vi "Encoder Config Pane.vi"(6 "_SubPanelMessages":refnum<notifier>, 9 "_myEmbeddedToFrameEvent":T5, 10 "_myEmbedded.Exit":refnum<user-event>, 11 "_Property Bundle":cluster{"Name":string, "Value":variant}[](array[cluster])) -> (1 "_Connection Informations":T1, 2 "_Scripter Input":T7)   [LabVIEW 2021]
doc: "Reads and decodes signals from an encoder. This Express VI reads the number of ticks that the encoder receives since the last counter reset."
uses:
  <vilib>/myRIO/Common/Express VI Framework/xctls/myRIO Channel Name/myRIO Channel Name.xctl
  <vilib>/myRIO/Common/Express VI Framework/typedefs/Config Pane to Framework Ref.ctl
  <vilib>/myRIO/Common/Express VI Framework/typedefs/Data Validate Ref.ctl
  <vilib>/myRIO/Common/Express VI Framework/typedefs/Scripter Input.ctl
  <vilib>/myRIO/Common/Express VI Framework/typedefs/WireThrough Terminal Names.ctl
  <vilib>/myRIO/Common/Express VI Framework/typedefs/Instrument Driver Method Descriptor Array.ctl
  <vilib>/myRIO/Common/Express VI Framework/typedefs/Instrument Driver Method Descriptor.ctl
  <vilib>/myRIO/Common/Express VI Framework/typedefs/Sub Panel Messages.ctl
  <vilib>/myRIO/Common/Express VI Framework/typedefs/Connection Informations.ctl
  <vilib>/myRIO/Common/Instrument Driver Framework/Utilities/typedefs/Channel Types.ctl
  <vilib>/myRIO/Common/Instrument Driver Framework/myRIO v1.0/Encoder/typedefs/Encoder Signal Mode.ctl
panel:
  in  "Encoder output signal type":enum32{"Quadrature phase", "Step and direction"}(radio) caption="Encoder output signal type:"
  out "_Channel Details:":string caption="Connections:"
  in  "Channel:":u16(xcontrol)
  in  "_Default Alias String":string
  in  "_VI Default Name (Edit and make value default)":string="Encoder"
  in  "Name:":string caption="Node name:"
  in  "_WireThrough Info (Edit and make value default)":T2={"WireThrough Top In"="Encoder Ref In", "WireThrough Bottom In"="error in (no error)", "WireThrough Top Out"="Encoder Ref Out", "WireThrough Bottom Out"="error out"}
  in  "_Template Array (Edit and make value default)":T3=[{"Function Name"="Smart Open", "VI Path"=path "<vilib>/myRIO/Instrument Drivers/Onboard IO/Encoder/vis", "Script"=TRUE, "Inputs"=[{"name"="Channel Name", "value"=variant, "Config Pane Only"=TRUE, "Build Array"=FALSE, "Bundle Cluster"=FALSE, "Show Term"=FALSE, "alias"=[], "Required Input"=FALSE}, {"name"="Encoder Signal Mode", "value"=variant, "Config Pane Only"=TRUE, "Build Array"=FALSE, "Bundle Cluster"=FALSE, "Show Term"=FALSE, "alias"=[], "Required Input"=FALSE}, {"name"="Start Counter", "value"=variant, "Config Pane Only"=TRUE, "Build Array"=FALSE, "Bundle Cluster"=FALSE, "Show Term"=FALSE, "alias"=[], "Required Input"=FALSE}], "Outputs"=[], "VI Class"=enum."Open", "Controls Refs[]"=[], "Inline"=FALSE}, {"Function Name"="Open", "VI Path"=path "<vilib>/myRIO/Instrument Drivers/Onboard IO/Encoder/vis", "Script"=FALSE, "Inputs"=[{"name"="Channel Name", "value"=variant, "Config Pane Only"=TRUE, "Build Array"=FALSE, "Bundle Cluster"=FALSE, "Show Term"=FALSE, "alias"=[], "Required Input"=FALSE}, {"name"="Encoder Signal Mode", "value"=variant, "Config Pane Only"=TRUE, "Build Array"=FALSE, "Bundle Cluster"=FALSE, "Show Term"=FALSE, "alias"=[], "Required Input"=FALSE}, {"name"="Start Counter", "value"=variant, "Config Pane Only"=TRUE, "Build Array"=FALSE, "Bundle Cluster"=FALSE, "Show Term"=FALSE, "alias"=[], "Required Input"=FALSE}], "Outputs"=[], "VI Class"=enum."Open", "Controls Refs[]"=[], "Inline"=FALSE}, {"Function Name"="Read", "VI Path"=path "<vilib>/myRIO/Instrument Drivers/Onboard IO/Encoder/vis", "Script"=TRUE, "Inputs"=[{"name"="Reset Counter", "value"=variant, "Config Pane Only"=FALSE, "Build Array"=FALSE, "Bundle Cluster"=FALSE, "Show Term"=TRUE, "alias"=[], "Required Input"=FALSE}], "Outputs"=[{"name"="Counter Value", "value"=variant, "Show Term"=TRUE, "Index Array"=FALSE, "Unbundle Cluster"=FALSE, "alias"=[]}, {"name"="Counter Direction", "value"=variant, "Show Term"=TRUE, "Index Array"=FALSE, "Unbundle Cluster"=FALSE, "alias"=[]}, {"name"="Overflow?", "value"=variant, "Show Term"=TRUE, "Index Array"=FALSE, "Unbundle Cluster"=FALSE, "alias"=[]}], "VI Class"=enum."Data", "Controls Refs[]"=[], "Inline"=FALSE}, {"Function Name"="Close", "VI Path"=path "<vilib>/myRIO/Instrument Drivers/Onboard IO/Encoder/vis", "Script"=FALSE, "Inputs"=[], "Outputs"=[], "VI Class"=enum."Close", "Controls Refs[]"=[], "Inline"=FALSE}]
  in  "_Test Close":bool
  # "User Visible Area"
  # "NOTE: Tab Order has been set\nfor this Front Panel.\n\nSee Edit>>Set Tabbing Order...\n\nAll controls that are not visible at \nruntime are excluded from Tabbing order\n\nTo exlude a control from context\nhelp prefix its label text with a '-'"
  # "Most encoders generate a quadrature phase signal that can be interpreted as Gray code. Choose this option if you are not sure about the signal type of your encoder."
  # "In some cases, encoders generate a signal for step and a signal for direction."
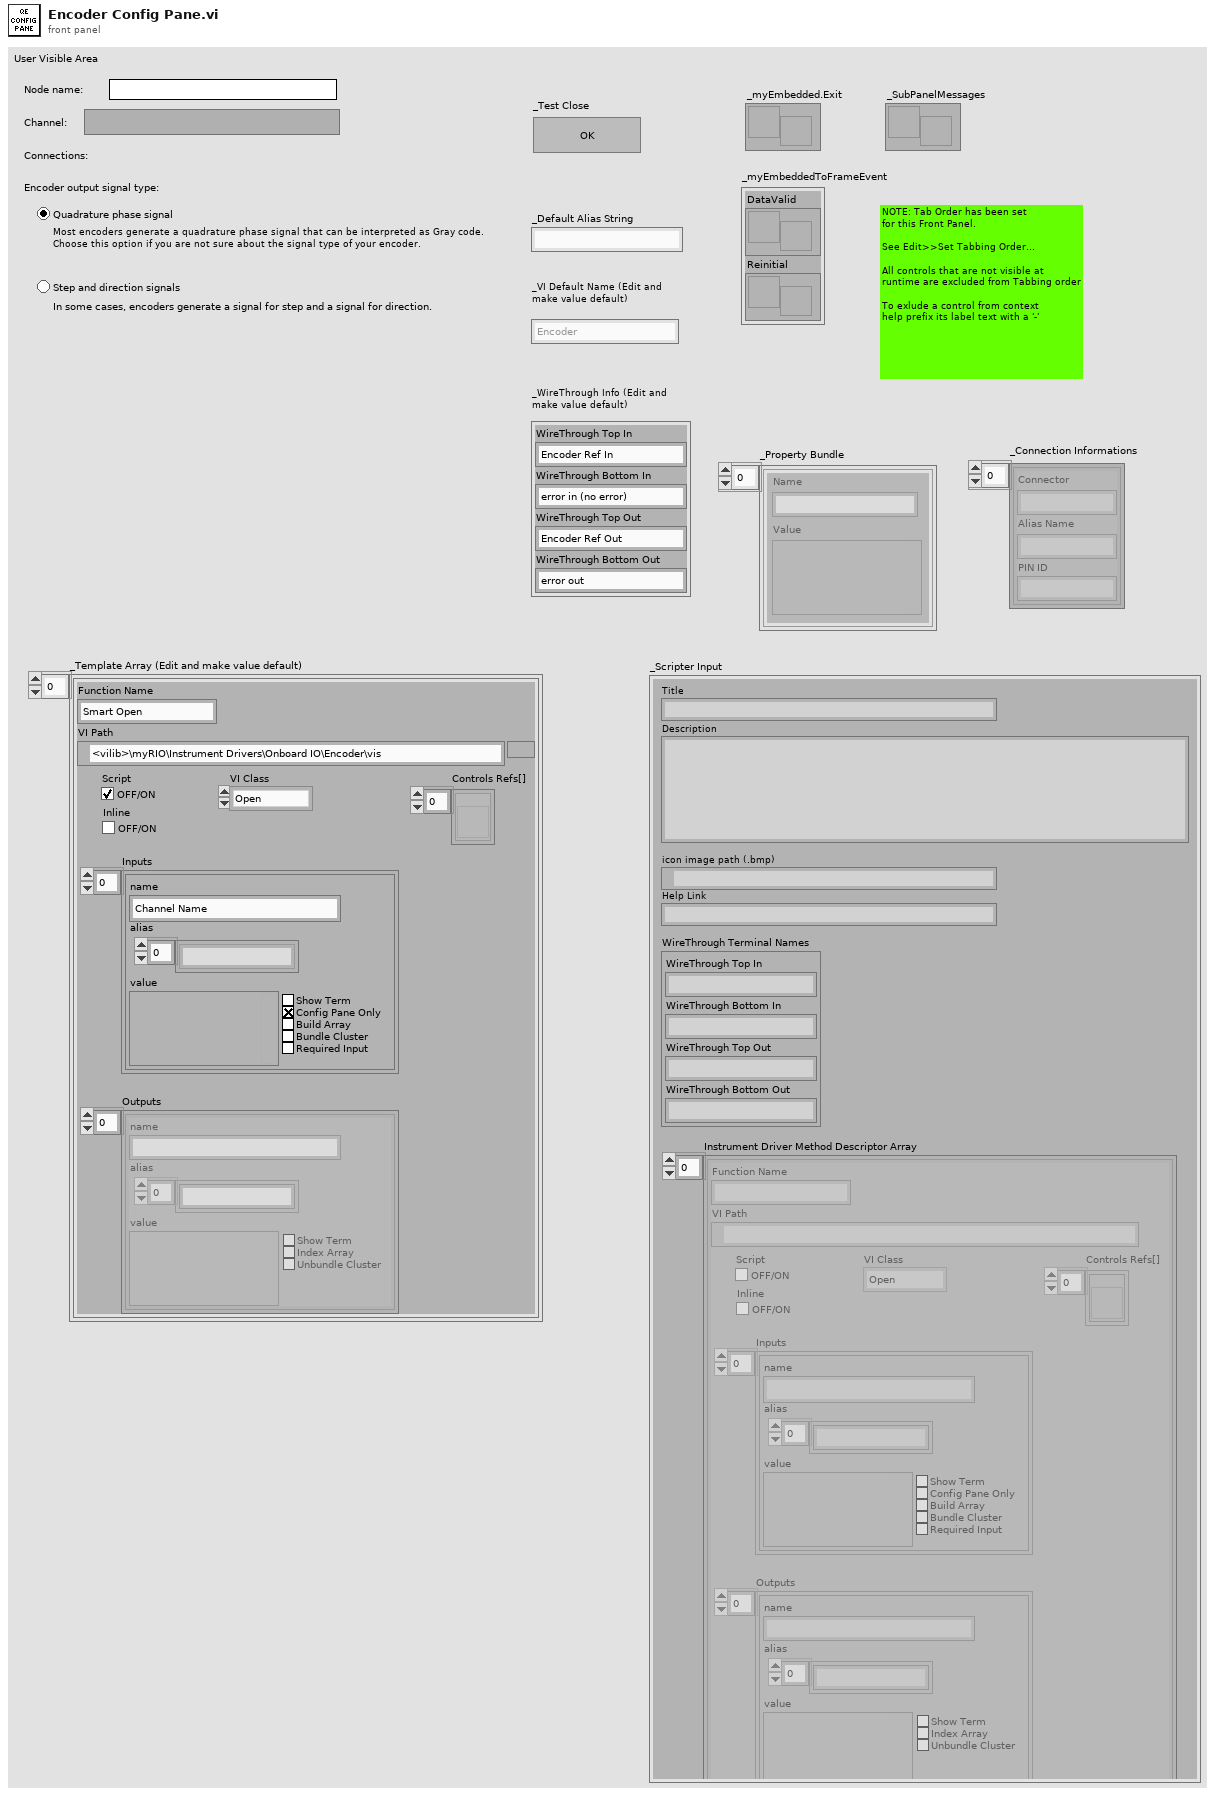
[diagram p1: front panel]
types:
  T1 = typedef "Connection Informations.ctl" = cluster{"Connector":string, "Alias Name":string, "PIN ID":string}[]
  T2 = typedef "WireThrough Terminal Names.ctl" = cluster{"WireThrough Top In":string, "WireThrough Bottom In":string, "WireThrough Top Out":string, "WireThrough Bottom Out":string}
  T3 = typedef "Instrument Driver Method Descriptor Array.ctl" = T4[]
  T4 = typedef "Instrument Driver Method Descriptor.ctl" = cluster{"Function Name":string, "VI Path":path, "Script":bool, "Inputs":cluster{"name":string, "value":variant, "Config Pane Only":bool, "Build Array":bool, "Bundle Cluster":bool, "Show Term":bool, "alias":string[], "Required Input":bool}[], "Outputs":cluster{"name":string, "value":variant, "Show Term":bool, "Index Array":bool, "Unbundle Cluster":bool, "alias":string[]}[], "VI Class":enum16{"Open", "Configure", "Data", "Manage", "Close"}, "Controls Refs[]":refnum<vi>[], "Inline":bool}
  T5 = typedef "Config Pane to Framework Ref.ctl" = cluster{"DataValid":T6, "Reinitial":refnum<user-event>}
  T6 = typedef "Data Validate Ref.ctl" = refnum<user-event>
  T7 = typedef "Scripter Input.ctl" = cluster{"Title":string, "Description":string, "icon image path (.bmp)":path, "Help Link":string, "WireThrough Terminal Names":T2, "Instrument Driver Method Descriptor Array":T3}
  T8 = typedef "Channel Types.ctl" = enum32{"Unknown", "AI", "AO", "DIO - DI", "DIO", "DIO - DO", "I2C", "PWM", "Encoder", "SPI", "UART", "Accelerometer", "DIO - LED", "DIO - Button", "AI (N Samples)", "AudioIn (N Samples)", "AO (N Samples)", "AudioOut (N Samples)", "DI (N Samples)", "DO (N Samples)", "AI IRQ", "DI IRQ", "Timer IRQ", "RSL", "Relay", "CAN", "AI (Continuous)", "AO (Continuous)"}
  T9 = typedef "Channel Info.ctl" = cluster{"Channel Name":string, "Alias":string, "Used?":bool, "Not Support?":bool, "Property Bundle":cluster{"Name":string, "Value":variant}[]}
  T10 = typedef "Sub Panel Messages.ctl" = enum16{"Initialized"}
  T11 = cluster{"Connector":string, "Alias Name":string, "PIN ID":string}
  T12 = typedef "Encoder Signal Mode.ctl" = enum16{"Quadrature phase signal", "Step and direction signal"}
  T13 = cluster{"name":string, "value":variant, "Config Pane Only":bool, "Build Array":bool, "Bundle Cluster":bool, "Show Term":bool, "alias":string[], "Required Input":bool}[]
  T14 = cluster{"name":string, "value":variant, "Config Pane Only":bool, "Build Array":bool, "Bundle Cluster":bool, "Show Term":bool, "alias":string[], "Required Input":bool}
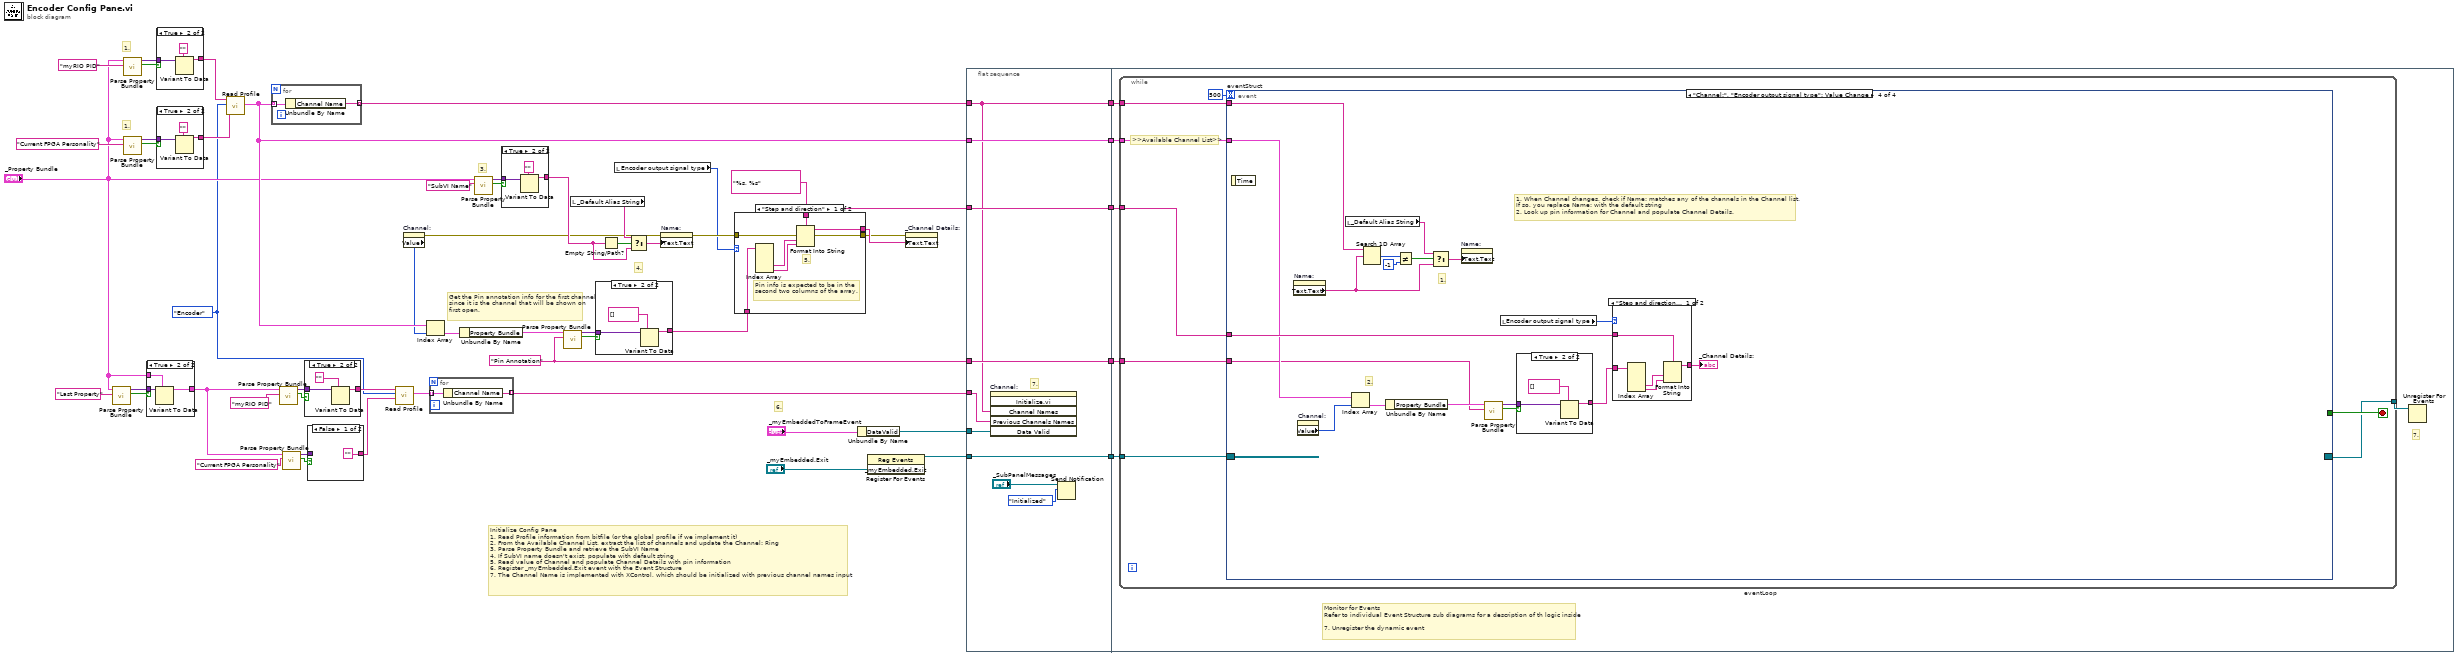
[diagram p0: block diagram]
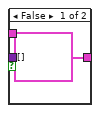
[diagram p2: hidden frame]
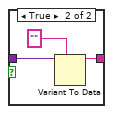
[diagram p3: hidden frame]
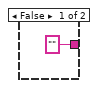
[diagram p4: hidden frame]
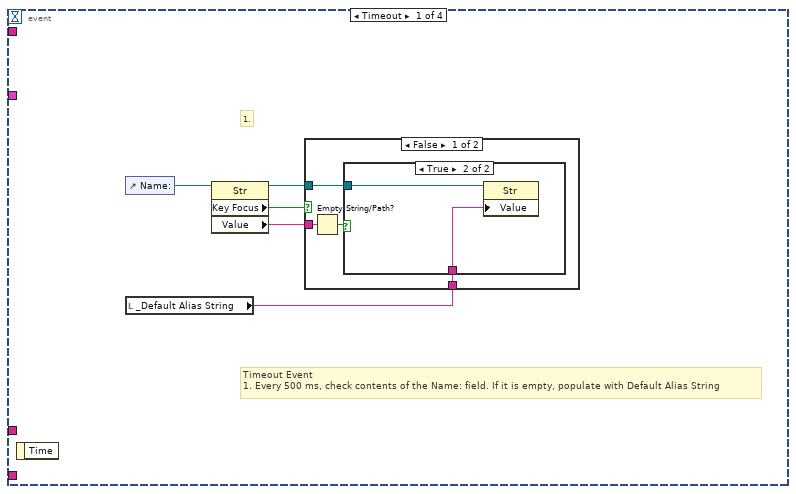
[diagram p5: hidden frame]
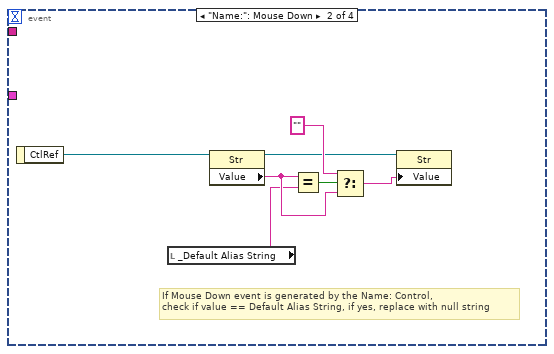
[diagram p8: hidden frame]
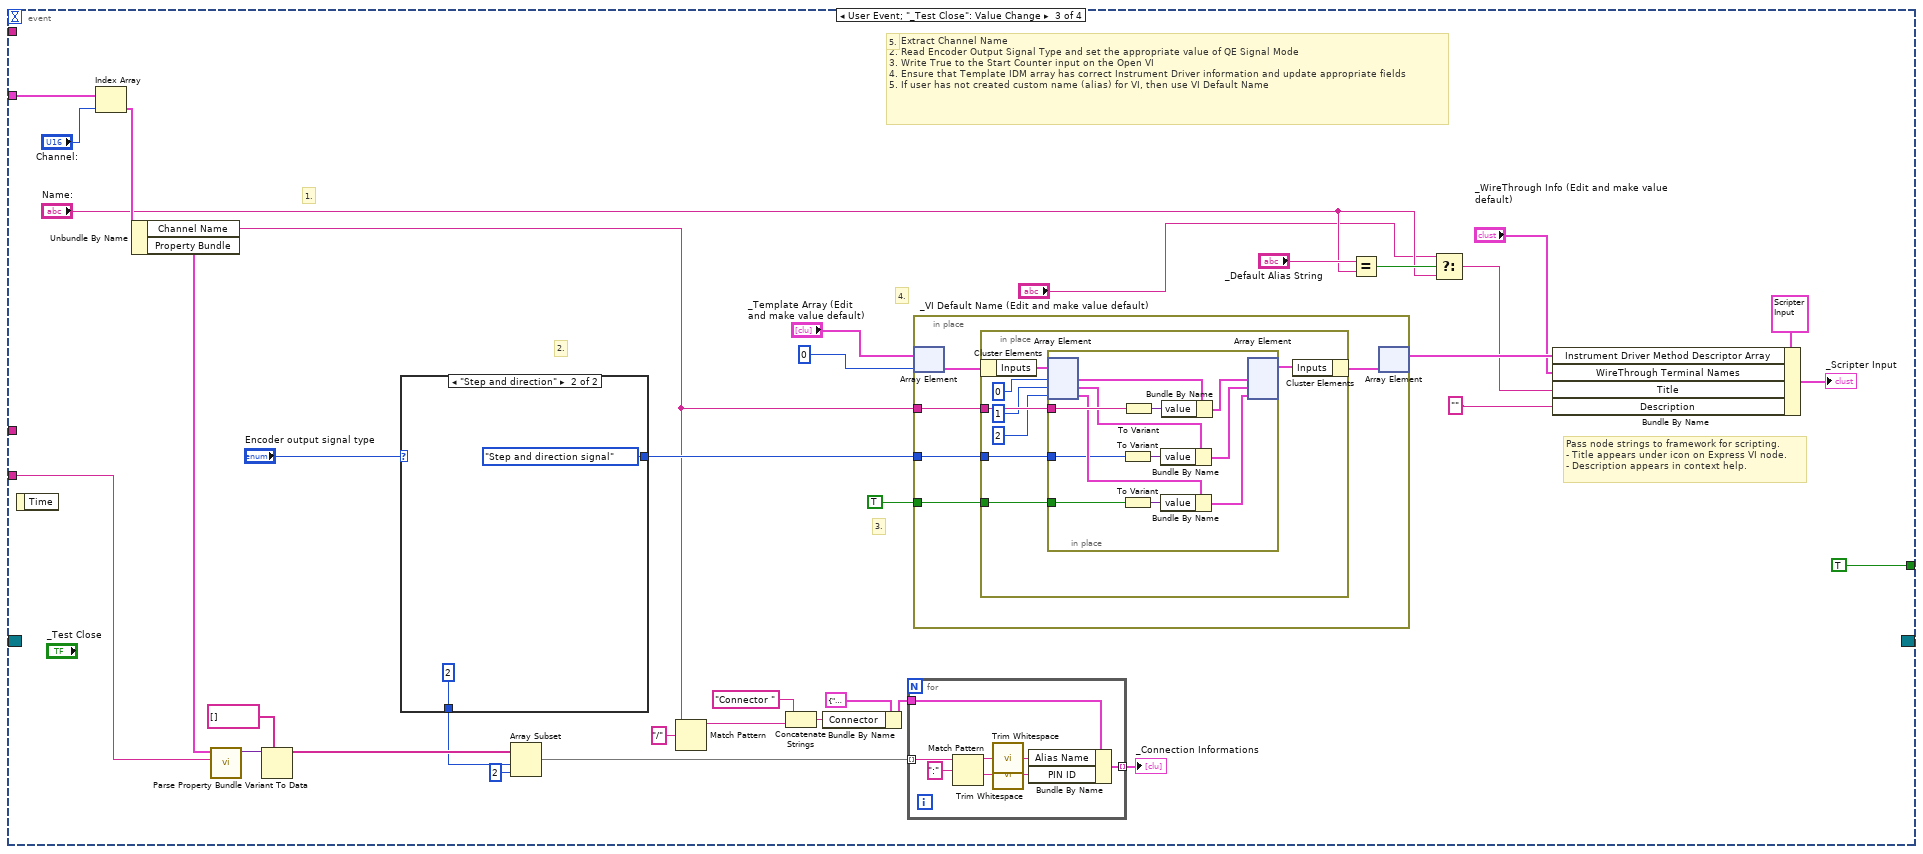
[diagram p9: hidden frame]
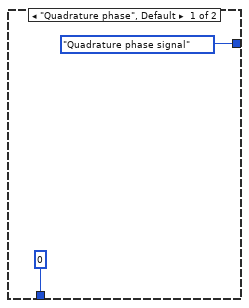
[diagram p10: hidden frame]
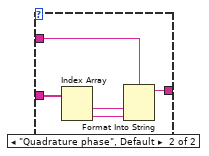
[diagram p11: hidden frame]
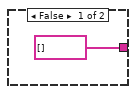
[diagram p12: hidden frame]
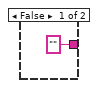
[diagram p13: hidden frame]
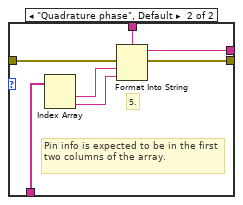
[diagram p14: hidden frame]
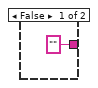
[diagram p15: hidden frame]
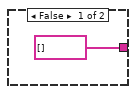
[diagram p16: hidden frame]
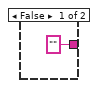
[diagram p17: hidden frame]
diagram:
  w1 = Channel_Types."Encoder" ("Channel to Read")
  w34 = "Pin Annotation" ("Name")
  w41 = "%s, %s"
  # "1."
  # "Get the Pin annotation info for the first channel  since it is the channel that will be shown on first open."
  # "1."
  # "6."
  # "4."
  # "3."
  # "Initialize Config Pane\n1. Read Profile information from bitfile (or the global profile if we implement it)\n2. From the Available Channel List, extract the list of channels and update the Channel: Ring\n3. Parse Property Bundle and retrieve the SubVI Name\n4. If SubVI name doesn't exist, populate with default string\n5. Read value of Channel and populate Channel Details with pin information \n6. Register _myEmbedded.Exit event with the Event Structure\n7. The Channel Name is implemented with XControl, which should be initialized with previous channel names input"
  n1 = call <vilib>:"Parse Property Bundle.vi"("Name"="Last Property", "Property Bundle"="_Property Bundle") -> ("Found?"=w8:bool, "Value"=w9:variant)  [unwired: 8 in]
  n2 = call <vilib>:"Parse Property Bundle.vi"("Name"="myRIO PID", "Property Bundle"="_Property Bundle") -> ("Found?"=w33:bool, "Value"=w32:variant)  [unwired: 8 in]
  n3 = call <vilib>:"Parse Property Bundle.vi"("Name"="Current FPGA Personality", "Property Bundle"="_Property Bundle") -> ("Found?"=w26:bool, "Value"=w27:variant)  [unwired: 8 in]
  n4 = case shown="True" w8 {
    tunnel: w9 -> [_ w59]
    tunnel: [cluster{"Name":string, "Value":variant}[] [] ("_Property Bundle") w58] -> w7
    tunnel: "_Property Bundle" -> [_ w57]
    frame False {
    }
    frame True {
      n5 = Variant To Data(type=w57, Variant=w59) -> (data=w58:cluster{"Name":string, "Value":variant}[])  [unwired: 1 in, 1 out]
    }
  }
  n6 = case shown="True" w33 {
    tunnel: w32 -> [_ w63]
    tunnel: ["" ("Name") w61] -> w30
    frame False {
    }
    frame True {
      n7 = Variant To Data(type="" ("Name"), Variant=w63) -> (data=w61:string)  [unwired: 1 in, 1 out]
    }
  }
  n8 = case shown="True" w26 {
    tunnel: w27 -> [_ w67]
    tunnel: ["" ("Name") w65] -> w25
    frame False {
    }
    frame True {
      n9 = Variant To Data(type="" ("Name"), Variant=w67) -> (data=w65:string)  [unwired: 1 in, 1 out]
    }
  }
  n10 = call <vilib>:"Read Profile.vi"("FPGA Name"=w25, "Channel to Read"=w1, "myRIO PID"=w30) -> ("Channel List Out"=w38:T9[])  [unwired: 7 in, 1 out]
  n11 = for {
    tunnel: [w69] -> w4 mode=indexing
    tunnel: w38 -> [w68] mode=indexing
    n12 = Unbundle By Name(w68) -> ("Channel Name"=w69:string)
  }
  n13 = call <vilib>:"Parse Property Bundle.vi"("Name"="myRIO PID", "Property Bundle"=w7) -> ("Found?"=w17:bool, "Value"=w16:variant)  [unwired: 8 in]
  n14 = call <vilib>:"Parse Property Bundle.vi"("Name"="Current FPGA Personality", "Property Bundle"=w7) -> ("Found?"=w12:bool, "Value"=w13:variant)  [unwired: 8 in]
  n15 = case shown="True" w17 {
    tunnel: w16 -> [_ w73]
    tunnel: ["" ("Name") w71] -> w18
    frame False {
    }
    frame True {
      n16 = Variant To Data(type="" ("Name"), Variant=w73) -> (data=w71:string)  [unwired: 1 in, 1 out]
    }
  }
  n17 = case shown="False" w12 {
    tunnel: w13 -> [_ w77]
    tunnel: ["" ("Name") w75] -> w11
    frame False {
    }
    frame True {
      n18 = Variant To Data(type="" ("Name"), Variant=w77) -> (data=w75:string)  [unwired: 1 in, 1 out]
    }
  }
  n19 = call <vilib>:"Read Profile.vi"("FPGA Name"=w11, "Channel to Read"=w1, "myRIO PID"=w18) -> ("Channel List Out"=w6:T9[])  [unwired: 7 in, 1 out]
  n20 = property on="Channel:" class="myRIO Channel Name (strict)"() -> (error out=w46:errorcluster, "Value"=w24:u16)  [unwired: 2 in, 1 out]
  n21 = Index Array(array=w38, index=w24) -> (element=w37:T9)
  n22 = for {
    tunnel: [w79] -> w2 mode=indexing
    tunnel: w6 -> [w78] mode=indexing
    n23 = Unbundle By Name(w78) -> ("Channel Name"=w79:string)
  }
  n24 = Unbundle By Name(w37) -> ("Property Bundle"=w36:cluster{"Name":string, "Value":variant}[])
  n25 = call <vilib>:"Parse Property Bundle.vi"("Name"="SubVI Name", "Property Bundle"="_Property Bundle") -> ("Found?"=w49:bool, "Value"=w48:variant)  [unwired: 8 in]
  n26 = case shown="True" w49 {
    tunnel: w48 -> [_ w83]
    tunnel: ["" ("Name") w81] -> w47
    frame False {
    }
    frame True {
      n27 = Variant To Data(type="" ("Name"), Variant=w83) -> (data=w81:string)  [unwired: 1 in, 1 out]
    }
  }
  n28 = call <vilib>:"Parse Property Bundle.vi"("Name"=w34, "Property Bundle"=w36) -> ("Found?"=w39:bool, "Value"=w40:variant)  [unwired: 8 in]
  n29 = local read "_Default Alias String"() -> (w51:string)
  n30 = case shown="True" w39 {
    tunnel: w40 -> [_ w87]
    tunnel: [string[] [] w86] -> w35
    frame False {
    }
    frame True {
      n31 = Variant To Data(type=string[] [], Variant=w87) -> (data=w86:string[])  [unwired: 1 in, 1 out]
    }
  }
  n32 = Empty String/Path?(string/path=w47) -> (empty?=w53:bool)
  n33 = local read "Encoder output signal type"() -> (w29:enum32{"Quadrature phase", "Step and direction"})
  n34 = Select(t=w51, s=w53, f=w47) -> (s? t:f=w52:string)
  n35 = property on="Name:" class="Str"(error in=w46, "Text.Text"=w52) -> (error out=w45:errorcluster)  [unwired: 1 in, 1 out]
  n36 = case shown="\"Step and direction\"" w29 {
    tunnel: w45 -> [w94 w101]
    tunnel: [w93 w100] -> w44
    tunnel: [w92 w99] -> w43
    tunnel: w41 -> [w91 w98]
    tunnel: w35 -> [w90 w95]
    frame "Step and direction" {
      # "Pin info is expected to be in the second two columns of the array."
      # "5."
      n37 = Index Array(array=w90) -> (element #3=w89:string, element #4=w88:string)  [unwired: 4 in, 2 out]
      n38 = Format Into String(format string=w91, error in=w94, w89, w88) -> (resulting string=w93:string, error out=w92:errorcluster)  [unwired: 1 in]
    }
    frame "Quadrature phase", Default {
      # "Pin info is expected to be in the first two columns of the array."
      # "5."
      n39 = Index Array(array=w95) -> (element #1=w97:string, element #2=w96:string)  [unwired: 2 in]
      n40 = Format Into String(format string=w98, error in=w101, w97, w96) -> (resulting string=w100:string, error out=w99:errorcluster)  [unwired: 1 in]
    }
  }
  n41 = Unbundle By Name("_myEmbeddedToFrameEvent") -> ("DataValid"=w23:T6)
  n42 = register-events("_myEmbedded.Exit") -> (reference out=w55:refnum<event-registration>)  [unwired: 2 in, 1 out]
  n43 = property on="_Channel Details:" class="Str"(error in=w43, "Text.Text"=w44) -> ()  [unwired: 1 in, 2 out]
  n44 = flat-sequence {
    tunnel: w23 -> [w104]
    tunnel: w34 -> [w107]
    tunnel: w38 -> [w108]
    tunnel: w41 -> [w109]
    tunnel: w55 -> [w110]
    tunnel: [w110] -> w22
    tunnel: [w109] -> w21
    tunnel: [w108] -> w20
    tunnel: [w107] -> w19
    tunnel: w4 -> [w103]
    tunnel: [w103] -> w3
    tunnel: w2 -> [w102]
    tunnel: w22 -> [w116]
    tunnel: w21 -> [w114]
    tunnel: w20 -> [w113]
    tunnel: w19 -> [w112]
    tunnel: w3 -> [w111]
    frame #0 {
      # "7."
      n45 = invoke on="Channel:" class="myRIO Channel Name (strict)" method="Initialize.vi"("Channel Names"=w103, "Previous Channels Names"=w102, "Data Valid"=w104) -> ()  [unwired: 3 in, 6 out]
      n46 = Send Notification(notification=Sub_Panel_Messages."Initialized", notifier="_SubPanelMessages") -> ()  [unwired: 1 in, 2 out]
    }
    frame #1 {
      # "7."
      # "Monitor for Events\nRefer to individual Event Structure sub diagrams for a description of th logic inside\n\n7. Unregister the dynamic event"
      n47 = while "eventLoop" {
        tunnel: w116 -> [w123]
        tunnel: [w122] -> w115
        tunnel: w113 -> [w120]
        tunnel: w114 -> [w119]
        tunnel: w112 -> [w118]
        tunnel: w111 -> [w117]
        stop <- w124 stop-if-true
        # ">>Available Channel List>>"
        n48 = event "eventStruct" shown="[3] \"Channel:\", \"Encoder output signal type\": Value Change" {
          selector: w123 -> [_ _ _ _]
          dyn-events: [_ _ _ _] -> w122
          timeout: 500 -> [_ _ _ _]
          tunnel: [_ _ TRUE ("_Test Close") _] -> w124
          tunnel: w120 -> [_ _ w176 w220]
          tunnel: w119 -> [_ _ _ w225]
          tunnel: w118 -> [_ _ w157 w217]
          tunnel: w117 -> [_ _ _ w215]
          event Timeout {
            # "Timeout Event\n1. Every 500 ms, check contents of the Name: field. If it is empty, populate with Default Alias String"
            # "1."
            n49 = event-data() -> ()  [unwired: 1 in, 1 out]
            n50 = control-ref of="Name:"() -> (w127:refnum<vi>)
            n51 = local read "_Default Alias String"() -> (w125:string)
            n52 = property on="Property Node" class="Str"(reference=w127) -> (reference out=w126:refnum<vi>, "Key Focus"=w128:bool, "Value"=w129:string)  [unwired: 1 in, 1 out]
            n53 = case shown="False" w128 {
              tunnel: w129 -> [w133 _]
              tunnel: w126 -> [w131 _]
              tunnel: w125 -> [w130 _]
              frame False {
                n54 = Empty String/Path?(string/path=w133) -> (empty?=w132:bool)
                n55 = case shown="True" w132 {
                  tunnel: w131 -> [_ w135]
                  tunnel: w130 -> [_ w134]
                  frame False {
                  }
                  frame True {
                    n56 = property on="Property Node" class="Str"(reference=w135, "Value"=w134) -> ()  [unwired: 1 in, 2 out]
                  }
                }
              }
              frame True {
              }
            }
          }
          event "Name:": Mouse Down {
            # "If Mouse Down event is generated by the Name: Control,\ncheck if value == Default Alias String, if yes, replace with null string"
            n57 = event-data() -> ("CtlRef"=w142:refnum<vi>)  [unwired: 1 in]
            n58 = local read "_Default Alias String"() -> (w136:string)
            n59 = property class="Str"(reference=w142) -> (reference out=w138:refnum<vi>, "Value"=w137:string)  [unwired: 1 in, 1 out]
            n60 = Equal?(x=w137, y=w136) -> (x = y?=w141:bool)
            n61 = Select(t="", s=w141, f=w137) -> (s? t:f=w139:string)
            n62 = property class="Str"(reference=w138, "Value"=w139) -> ()  [unwired: 1 in, 2 out]
          }
          event User Event; "_Test Close": Value Change {
            # "3."
            # "1."
            # "2."
            # "1. Extract Channel Name\n2. Read Encoder Output Signal Type and set the appropriate value of QE Signal Mode \n3. Write True to the Start Counter input on the Open VI \n4. Ensure that Template IDM array has correct Instrument Driver information and update appropriate fields\n5. If user has not created custom name (alias) for VI, then use VI Default Name"
            # "5."
            # "4."
            # "Pass node strings to framework for scripting.\n- Title appears under icon on Express VI node.\n- Description appears in context help."
            n63 = event-data() -> ()  [unwired: 1 in, 1 out]
            n64 = Index Array(array=w176, index="Channel:") -> (element=w165:T9)
            n65 = Unbundle By Name(w165) -> ("Channel Name"=w152:string, "Property Bundle"=w158:cluster{"Name":string, "Value":variant}[])
            n66 = call <vilib>:"Parse Property Bundle.vi"("Name"=w157, "Property Bundle"=w158) -> ("Value"=w156:variant)  [unwired: 8 in, 1 out]
            n67 = Variant To Data(type=string[] [], Variant=w156) -> (data=w145:string[])  [unwired: 1 in, 1 out]
            n68 = case shown="\"Step and direction\"" "Encoder output signal type" {
              tunnel: [Encoder_Signal_Mode."Quadrature phase signal" ("QE Signal Mode") Encoder_Signal_Mode."Step and direction signal" ("QE Signal Mode")] -> w161
              tunnel: [0 ("index") 2 ("index")] -> w143
              frame "Quadrature phase", Default {
              }
              frame "Step and direction" {
              }
            }
            n69 = Array Subset(array=w145, index=w143, length=2) -> (w146:string[])
            n70 = Match Pattern(string=w152, regular expression="/") -> (before substring=w150:string)  [unwired: 1 in, 3 out]
            n71 = Concatenate Strings("Connector " ("string"), w150) -> (w148:string)
            n72 = Bundle By Name(cluster=T11 {"Connector"="", "Alias Name"="", "PIN ID"=""} ("Connection Information"), "Connector"=w148) -> (w153:T11)
            n73 = for {
              tunnel: w153 -> [w185]
              tunnel: [w181] -> w147 mode=indexing
              tunnel: w146 -> [w178] mode=indexing
              n74 = Match Pattern(string=w178, regular expression=":") -> (before substring=w183:string, after substring=w182:string)  [unwired: 1 in, 2 out]
              n75 = call <vilib>:"Trim Whitespace.vi"("string"=w183) -> ("trimmed string"=w180:string)  [unwired: 1 in]
              n76 = call <vilib>:"Trim Whitespace.vi"("string"=w182) -> ("trimmed string"=w179:string)  [unwired: 1 in]
              n77 = Bundle By Name(cluster=w185, "Alias Name"=w180, "PIN ID"=w179) -> (w181:T11)
            }
            "_Connection Informations" <- w147
            n78 = in-place {
              in-place-border: w152 -> [w192]
              in-place-border: w161 -> [w191]
              in-place-border: TRUE -> [w190]
              n79 = in-place-array #1("_Template Array (Edit and make value default)", 0) -> (w194:T4)
              n80 = in-place {
                in-place-border: w192 -> [w201]
                in-place-border: w191 -> [w196]
                in-place-border: w190 -> [w195]
                n81 = in-place-cluster #2(w194) -> ("Inputs"=w202:T13)
                n82 = in-place {
                  in-place-border: w201 -> [w211]
                  in-place-border: w196 -> [w206]
                  in-place-border: w195 -> [w205]
                  n83 = in-place-array #3(w202, 0, 1, 2) -> (w214:T14, w208:T14, w207:T14)
                  n84 = To Variant(anything=w206) -> (Variant=w210:variant)
                  n85 = To Variant(anything=w205) -> (Variant=w209:variant)
                  n86 = To Variant(anything=w211) -> (Variant=w212:variant)
                  n87 = Bundle By Name(cluster=w208, "value"=w210) -> (w204:T14)
                  n88 = Bundle By Name(cluster=w207, "value"=w209) -> (w203:T14)
                  n89 = Bundle By Name(cluster=w214, "value"=w212) -> (w213:T14)
                  n90 = in-place-array #3(w213, w204, w203) -> (w200:T13)  [unwired: 3 out]
                }
                n91 = in-place-cluster #2("Inputs"=w200) -> (w193:T4)
              }
              n92 = in-place-array #1(w193) -> (w175:T3)  [unwired: 1 out]
            }
            n93 = Equal?(x="_Default Alias String", y="Name:") -> (x = y?=w167:bool)
            n94 = Select(t="_VI Default Name (Edit and make value default)", s=w167, f="Name:") -> (s? t:f=w166:string)
            n95 = Bundle By Name(cluster=T7 {"Title"="", "Description"="", "icon image path (.bmp)"=path "", "Help Link"="", "WireThrough Terminal Names"={"WireThrough Top In"="", "WireThrough Bottom In"="", "WireThrough Top Out"="", "WireThrough Bottom Out"=""}, "Instrument Driver Method Descriptor Array"=[]} ("Scripter Input"), "Instrument Driver Method Descriptor Array"=w175, "WireThrough Terminal Names"="_WireThrough Info (Edit and make value default)", "Title"=w166, "Description"="" ("Title")) -> (→"_Scripter Input":T7)
          }
          event "Channel:", "Encoder output signal type": Value Change {
            # "1. When Channel changes, check if Name: matches any of the channels in the Channel list. \nIf so, you replace Name: with the default string\n2. Look up pin information for Channel and populate Channel Details."
            # "2."
            # "1."
            n96 = event-data() -> ()  [unwired: 1 in, 1 out]
            n97 = property on="Name:" class="Str"() -> ("Text.Text"=w229:string)  [unwired: 2 in, 2 out]
            n98 = property on="Channel:" class="myRIO Channel Name (strict)"() -> ("Value"=w219:u16)  [unwired: 2 in, 2 out]
            n99 = local read "_Default Alias String"() -> (w227:string)
            n100 = Index Array(array=w220, index=w219) -> (element=w222:T9)
            n101 = Search 1D Array(1D array=w215, element=w229) -> (index of element=w232:i32)  [unwired: 1 in]
            n102 = Unbundle By Name(w222) -> ("Property Bundle"=w221:cluster{"Name":string, "Value":variant}[])
            n103 = Not Equal?(x=w232, y=-1) -> (x != y?=w230:bool)
            n104 = Select(t=w227, s=w230, f=w229) -> (s? t:f=w228:string)
            n105 = property on="Name:" class="Str"("Text.Text"=w228) -> ()  [unwired: 2 in, 2 out]
            n106 = call <vilib>:"Parse Property Bundle.vi"("Name"=w217, "Property Bundle"=w221) -> ("Found?"=w223:bool, "Value"=w224:variant)  [unwired: 8 in]
            n107 = local read "Encoder output signal type"() -> (w216:enum32{"Quadrature phase", "Step and direction"})
            n108 = case shown="True" w223 {
              tunnel: w224 -> [_ w246]
              tunnel: [string[] [] w245] -> w218
              frame False {
              }
              frame True {
                n109 = Variant To Data(type=string[] [], Variant=w246) -> (data=w245:string[])  [unwired: 1 in, 1 out]
              }
            }
            n110 = case shown="\"Step and direction\"" w216 {
              tunnel: [w237 w242] -> w226
              tunnel: w225 -> [w236 w241]
              tunnel: w218 -> [w235 w238]
              frame "Step and direction" {
                n111 = Index Array(array=w235) -> (element #3=w234:string, element #4=w233:string)  [unwired: 4 in, 2 out]
                n112 = Format Into String(format string=w236, w234, w233) -> (resulting string=w237:string)  [unwired: 2 in, 1 out]
              }
              frame "Quadrature phase", Default {
                n113 = Index Array(array=w238) -> (element #1=w240:string, element #2=w239:string)  [unwired: 2 in]
                n114 = Format Into String(format string=w241, w240, w239) -> (resulting string=w242:string)  [unwired: 2 in, 1 out]
              }
            }
            "_Channel Details:" <- w226
          }
        }
      }
      n115 = Unregister For Events(event registration refnum=w115) -> ()  [unwired: 1 in, 1 out]
    }
  }
